vi "Array_sum.vi"(10 "Array":dbl[](array[numeric])) -> (2 "Numeric":dbl)   [LabVIEW 2021]
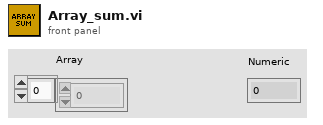
[diagram p1: front panel]
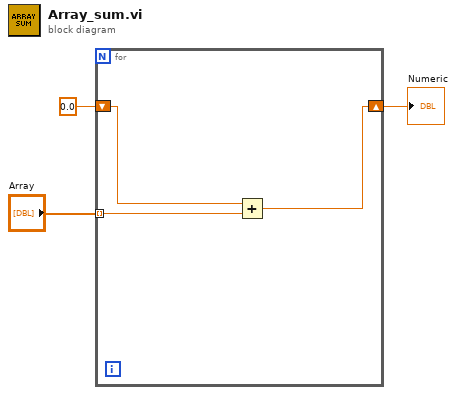
[diagram p0: block diagram]
diagram:
  n1 = for {
    tunnel: "Array" -> [w6] mode=indexing
    shift-right: [w4] -> w1
    shift-left: 0.0 -> [w5]
    n2 = Add(x=w5, y=w6) -> (x+y=w4:dbl)
  }
  "Numeric" <- w1
